vi "New Basic Subscription.vi"(10 "Ignore Past Updates? (F)":bool, 11 "BasicSubscription In":refnum<class "BasicSubscription.lvclass">) -> (3 "BasicSubscription Out":refnum<class "BasicSubscription.lvclass">)   [LabVIEW 2020, in "SubscriptionPolicy.lvlib" / "BasicSubscription.lvclass"]
doc: "新建基本订阅"
uses:
  BasicSubscription.lvclass
  BasicSubscription.lvclass/BasicSubscription.ctl
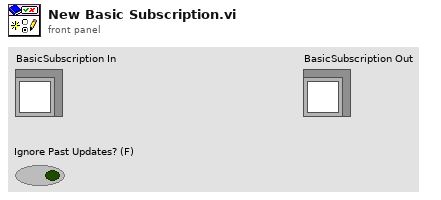
[diagram p1: front panel]
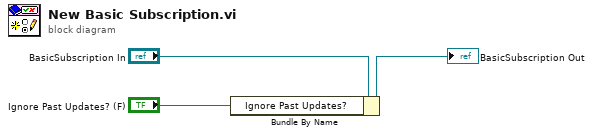
[diagram p0: block diagram]
diagram:
  n1 = Bundle By Name(cluster="BasicSubscription In", "Ignore Past Updates?"="Ignore Past Updates? (F)") -> (→"BasicSubscription Out":refnum<class "BasicSubscription.lvclass">)
